vi "Clear.vi"(8 "error in (no error)":errorcluster, 11 "Dictionary in":refnum<class "Dictionary.lvclass">) -> (0 "error out":errorcluster, 3 "Dictionary out":refnum<class "Dictionary.lvclass">)   [LabVIEW 2018, in "Application.lvlib" / "Dictionary.lvclass"]
uses:
  Dictionary.lvclass
  Dictionary.lvclass/Dictionary.ctl
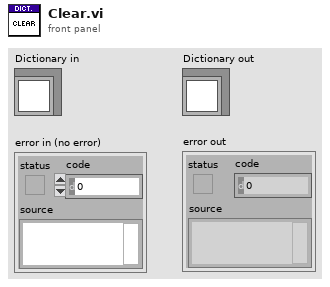
[diagram p1: front panel]
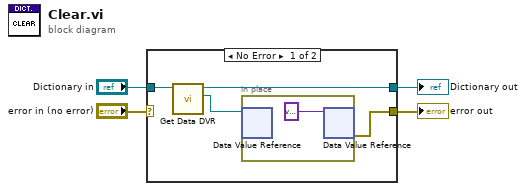
[diagram p0: block diagram]
diagram:
  n1 = case shown="No Error" "error in (no error)" {
    selector: "error in (no error)" -> [_ w11]
    tunnel: [w5 w11] -> w3
    tunnel: [w6 w10] -> w1
    tunnel: "Dictionary in" -> [w8 w10]
    frame No Error {
      n2 = call "Get Data DVR.vi"("Dictionary in"=w8) -> ("Data DVR"=w7:refnum<data-value>, "Dictionary out"=w6:refnum<class "Dictionary.lvclass">)  [unwired: 8 in, 1 out]
      n3 = in-place {
        n4 = in-place-dvr #1(w7) -> ()  [unwired: 2 out]
        n5 = in-place-dvr #1(variant ("data value")) -> (w5:errorcluster)  [unwired: 1 out]
      }
    }
    frame Error {
    }
  }
  "error out" <- w3
  "Dictionary out" <- w1
